vi "UseArrayOfClasses.vi"() -> (3 "output array":refnum<class "myClass.lvclass">[](array[class]))   [LabVIEW 2012]
uses:
  ClassDefinitions/SimpleClassWithProperties/myClass.lvclass
panel:
  in  "Array":refnum<class "myClass.lvclass">[](array[class])
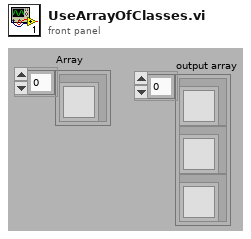
[diagram p1: front panel]
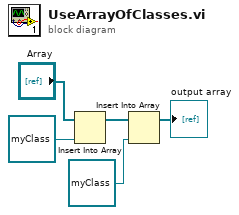
[diagram p0: block diagram]
diagram:
  n1 = Insert Into Array(array="Array", new element=refnum<class "myClass.lvclass"> refnum ("myClass.lvclass")) -> (w3:refnum<class "myClass.lvclass">[])  [unwired: 1 in]
  n2 = Insert Into Array(array=w3, new element=refnum<class "myClass.lvclass"> refnum ("myClass.lvclass")) -> (→"output array":refnum<class "myClass.lvclass">[])  [unwired: 1 in]
